vi "Stop Acquisition.vi"(8 "error in (no error)":errorcluster, 11 "Hardware Resources in":T1={"VISA resource name"="", "Mode (0: Normal) "=0, "Voltage"={"Element (0: All)"=0, "V Range (200)"=4}, "Current"={"A Range (2)"=7, "A Terminal (0: 5A)"=0, "Element (0: ALL)"=0}, "Observation Time"=10, "Modules on/off"={"Module 1"=FALSE, "Module 2"=FALSE, "Module 3"=FALSE, "Module 4"=FALSE}} {"Observation Time" items=["1ksec", "400sec", "200sec", "100sec", "40sec", "20sec", "10sec", "4sec", "2sec", "1sec", "400msec", "200msec", "100msec", "40msec", "20msec", "10msec", "4msec", "2msec", "1msec", "400usec", "200usec", "100usec", "40usec", "20usec", "10usec"]; "Mode (0: Normal)" items=["Normal", "Harmonics"]; "Current"."Element (0: ALL)" items=["All", "Element 1", "Element 2", "Element 3", "Element 4"]; "Current"."A Terminal (0: 5A)" items=["5A", "20A", "Sensor"]; "Current"."A Range (2)" items=["AUTO", "0.1", "0.2", "0.4", "1", "2", "4", "10", "20", "40", "100"]; "Voltage"."V Range (200)" items=["AUTO", "30", "60", "120", "200", "300", "600", "1200", "2000"]; "Voltage"."Element (0: All)" items=["All", "Element 1", "Element 2", "Element 3", "Element 4"]}) -> (0 "error out":errorcluster)   [LabVIEW 2013, in "YKPZ400 Acquisition.lvlib"]
doc: "Stops the acquisition."
uses:
  YKPZ400 Acquisition.lvlib
  Hardware Configuration.ctl
  <instrlib>/Yokogawa PZ4000/Yokogawa PZ4000.lvlib
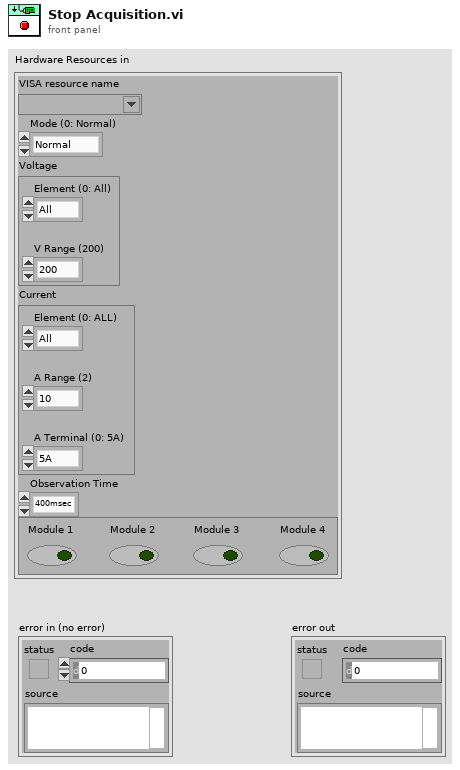
[diagram p1: front panel]
types:
  T1 = typedef "YKPZ400 Acquisition.lvlib/Hardware Configuration.ctl" = cluster{"VISA resource name":refnum<visa-resource-name>, "Mode (0: Normal) ":u16, "Voltage":cluster{"Element (0: All)":u16, "V Range (200)":u16}, "Current":cluster{"A Range (2)":u16, "A Terminal (0: 5A)":u16, "Element (0: ALL)":u16}, "Observation Time":u16, "Modules on/off":cluster{"Module 1":bool, "Module 2":bool, "Module 3":bool, "Module 4":bool}}
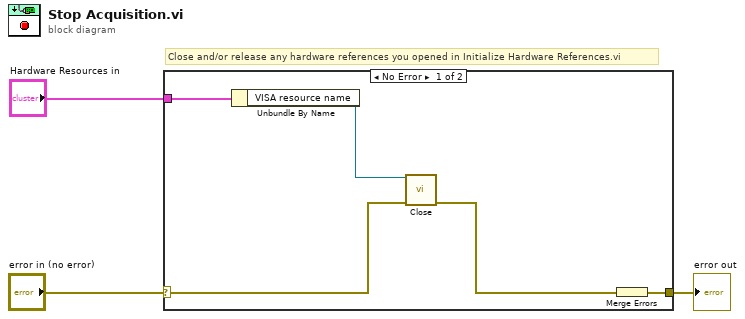
[diagram p0: block diagram]
diagram:
  # "Close and/or release any hardware references you opened in Initialize Hardware References.vi"
  n1 = case shown="No Error" "error in (no error)" {
    selector: "error in (no error)" -> [w5 w9]
    tunnel: [w8 w9] -> w2
    tunnel: "Hardware Resources in" -> [w7 _]
    frame No Error {
      n2 = Unbundle By Name(w7) -> ("VISA resource name"=w6:refnum<visa-resource-name>)
      n3 = call <instrlib>:"Close.vi"("VISA resource name"=w6, "error in (no error)"=w5) -> ("error out"=w4:errorcluster)  [unwired: 13 in]
      n4 = Merge Errors(w4) -> (w8:errorcluster)
    }
    frame Error {
    }
  }
  "error out" <- w2
